vi "ATE_spoldrx_cal_at_IF.vi"() -> ()   [LabVIEW 2012]
doc: "Use this template to build a producer/consumer design pattern with events to produce queue items. Use this design pattern instead of the User Interface Event Handler pattern for user interfaces when you want to execute code asynchronously in response to an event without slowing the user interface responsiveness."
uses:
  Rvp8PowerData.ctl
  <vilib>/Analysis/NI_AALPro.lvlib
panel:
  in  "ABORT":bool
  in  "READY":bool
  out "Instructions":string="rvp8 calibration vi\n\n1 - Disable or turn off transmitter\n2 - Stow Antenna (point vertically)\n3 - Start the labview program by clicking the Run arrow\n     (left most button under  drop down menues)\n     start cycle time about 35 seconds\n3 - Wait for the red 'BUSY' light to change to green 'READY'\n     The 'active' controls on the control tab are the 'TsPring/TsGrabber'\n     and the 'Start dBm', 'Step Size' and 'Steps' controls \n4 - Calibrate with the red  'Calibrate' button\n      calibration cycle time is about 5 minutes\n5 - Calibration cycle can be aborted with the 'Abort Cal' button which\n     is visable only during the cal cycle\n6 - exit the program with the red 'EXIT' button\n      exit cycle time about 20 seconds\n\nHints:\nWait for the green 'READY' light before clicking buttons"
  out "70dB\nAttenuators":bool[](array[boolean])
  out "70 Verfied":bool
  out "121dB\nAttenuators":bool[](array[boolean])
  out "121 Verified":bool
  in  "Configuration 1":bool
  out "Cal Output File":path
  out "Cal differences":cluster{dbl[], dbl[]}[](graph)
  out "drx calibration":cluster{dbl[], dbl[]}[](graph)
  out "Cal file name":string
  in  "Cal data directory":string="/home/spol/projDir/data/cal/ate/drx_cal"
  in  "Set SigGen":bool
  in  "Initialize":bool
  in  "70 dB":bool
  in  "121 dB":bool
  in  "Switches":bool
  in  "Calibrate":bool
  in  "Stop":bool
  in  "ATE TABS":enum32{"Status", "Controls"}(tab)=enum."Controls"
  out "ATE Switch Status":T1
  out "drx Power":T2 {"time" format="%<%H:%M:%S\n%Y/%m/%d>T"}
  out "Signal Generator Status":T3={"Frequency (GHz)"=0.0, "RF Power (dBm)"=0.0, "RF Power"=TRUE} {"RF Power (dBm)" format="%.2g"}
  in  "Start dBm":dbl=-14.0 min=-100.0 max=14.0 step=1.0
  in  "Steps":i32=64
  in  "Steps Size":dbl=2.0 min=0.1 max=10.0 step=0.1 format="%.1g"
  in  "121 dB Atten":i32=121 min=0 max=121 step=1
  in  "70 dB Attn":i32=70 min=0 max=70 step=10
  in  "ATE Switches":T4={"Reversing Switch"=enum."Normal Function", "IO Switch #1 Input"=enum."NONE", "IO Switch #1 Output"=enum."NONE", "IO Switch #2 Input"=enum."NONE", "IO Switch #2 Output"=enum."NONE", "Signal Out Input"=enum."NONE", "Signal Out Output"=enum."NONE", "Signal Source Input"=enum."NONE", "Signal Source Output"=enum."NONE", "Power Meter Switch Input"=enum."NONE", "Pouer Meter Switch Output"=enum."NONE", "Amplifier Switch"=enum."Include Amp"}
  out "P-State":string
  out "C-State":string
  in  "BUSY":bool
  # "ATE drx cal Program"
  # "10 dB"
  # "20 dB"
  # "40 dB"
  # "1 dB"
  # "2 dB"
  # "4 dB"
  # "4 dB"
  # "10 dB"
  # "20 dB"
  # "40 dB"
  # "40 dB"
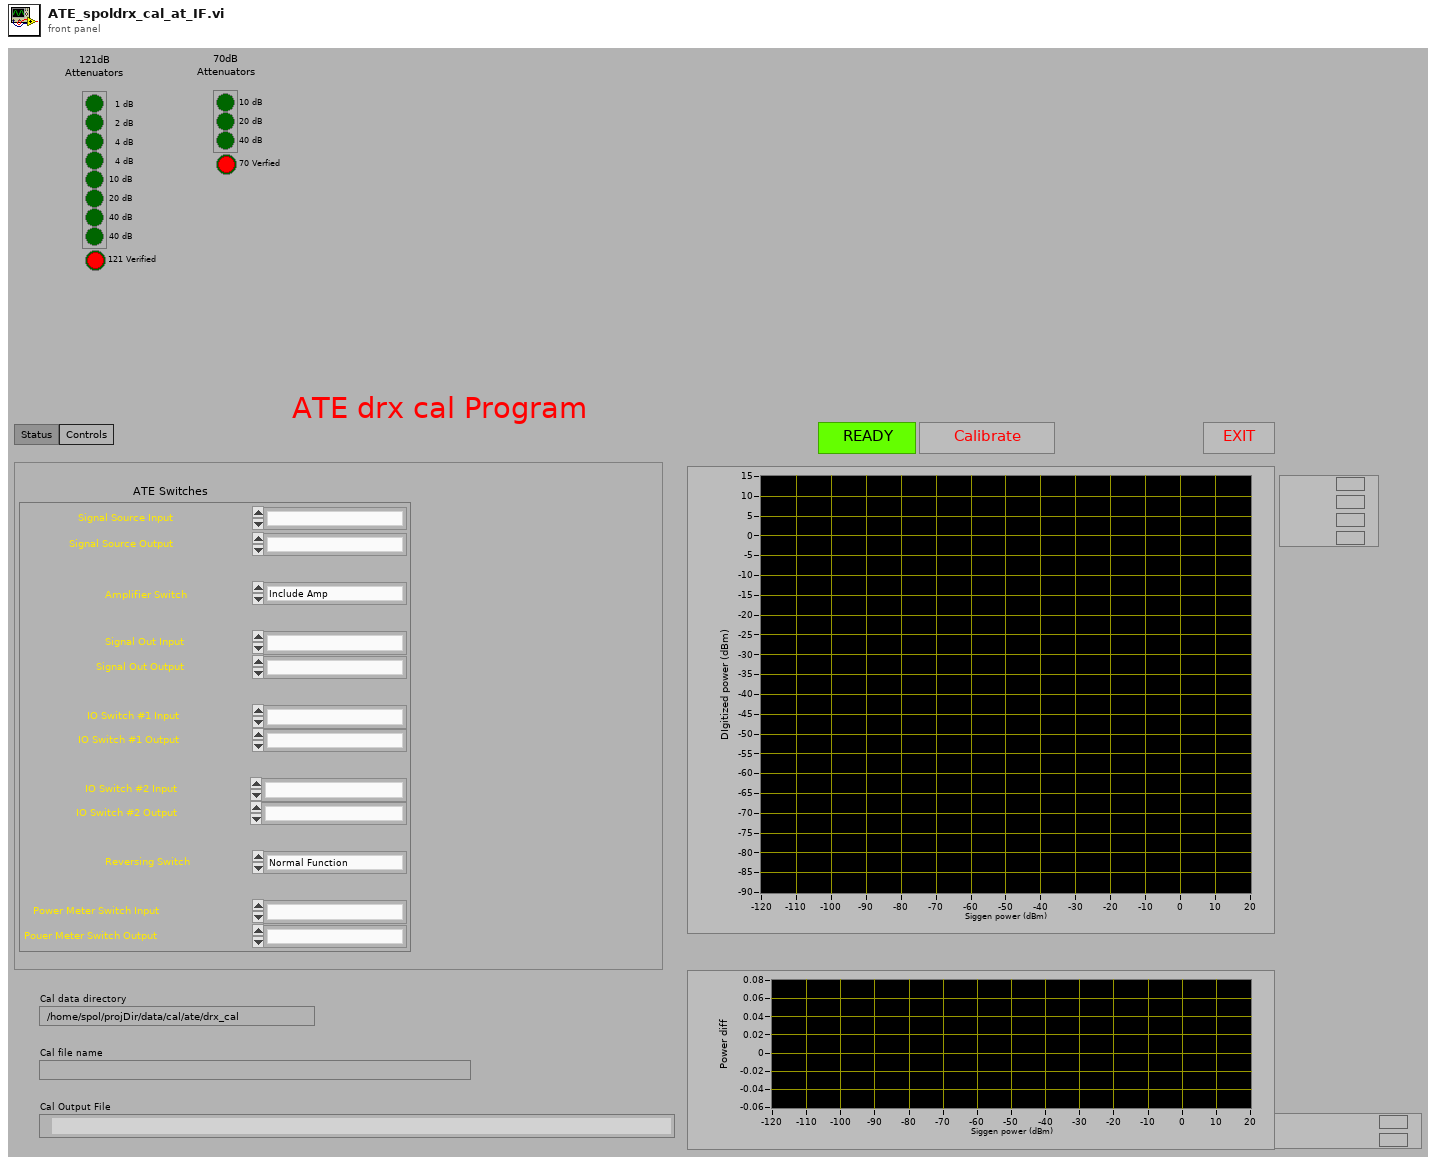
[diagram p1: front panel]
types:
  T1 = cluster{"Reversing Switch ":bool, "IO Switch #1":bool, "IO Switch #2":bool, "Signal Out":bool, "Signal Source":bool, "Power Meter":bool, "Amp By Pass":bool}
  T2 = typedef "Rvp8PowerData.ctl" = cluster{"success":bool, "time":dbl, "el":dbl, "az":dbl, "dbm0":dbl, "dbm1":dbl, "dbmHc":dbl, "dbmHx":dbl, "dbmVc":dbl, "dbmVx":dbl}
  T3 = cluster{"Frequency (GHz)":dbl, "RF Power (dBm)":dbl, "RF Power":bool}
  T4 = cluster{"Reversing Switch":enum16{"Normal Function", "Reversing Function"}, "IO Switch #1 Input":enum16{"NONE", "AHR (J2)", "Splitter", "Signal Out Switch (S3)", "Reversing Switch"}, "IO Switch #1 Output":enum16{"NONE", "AHR (J2)", "Delay Device (S4)", "Power Meter Switch (S5)", "Reversing Switch"}, "IO Switch #2 Input":enum16{"NONE", "AVR (J3)", "Splitter", "Signal Out Switch (S3)", " 2W Term (TM1)", "Reversing Switch"}, "IO Switch #2 Output":enum16{"NONE", "AVR (J3)", "Signal Out Switch (S3)", "Power Meter Switch (S5)", "Reversing Switch", "2W Term (TM1)"}, "Signal Out Input":enum16{"NONE", "Amp Bypass Switch (S6)", "IO Switch #1 (S1)", "IO Switch #2 (S2)", "2W Term (TM3)"}, "Signal Out Output":enum16{"NONE", "2 Watt Term (TM3)", "Splitter", "Power Meter Switch (S5)"}, "Signal Source Input":enum16{"NONE", "Delay Device", "Signal Generator (J7)", "Inside Noise Box NF (J5)", "2W Term (TM3)"}, "Signal Source Output":enum16{"NONE", "Amp Bypass Switch", "Test Pulse Generator", "Power Meter Switch (S5)"}, "Power Meter Switch Input":enum16{"NONE", "IO Switch #1 (S1)", "Signal Source Switch (S4)", "Signal Out Switch (S3)", "IO Switch #2 (S2)", "TXH-TXV Switch (J8)"}, "Pouer Meter Switch Output":enum16{"NONE", "Power Meter (J6)"}, "Amplifier Switch":enum16{"Bypass Amp", "Include Amp"}}
  T5 = cluster{"Frequency (GHz)":dbl, "RF Power (dBm)":dbl, "RF ON/OFF":bool}
  T6 = enum16{"open", "replace", "create", "open or create", "replace or create", "replace or create with confirmation"}
  T7 = typedef "drxPowerData.ctl" = cluster{"success":bool, "time":dbl, "el":dbl, "az":dbl, "dbm0":dbl, "dbm1":dbl, "dbmHc":dbl, "dbmHx":dbl, "dbmVc":dbl, "dbmVx":dbl}
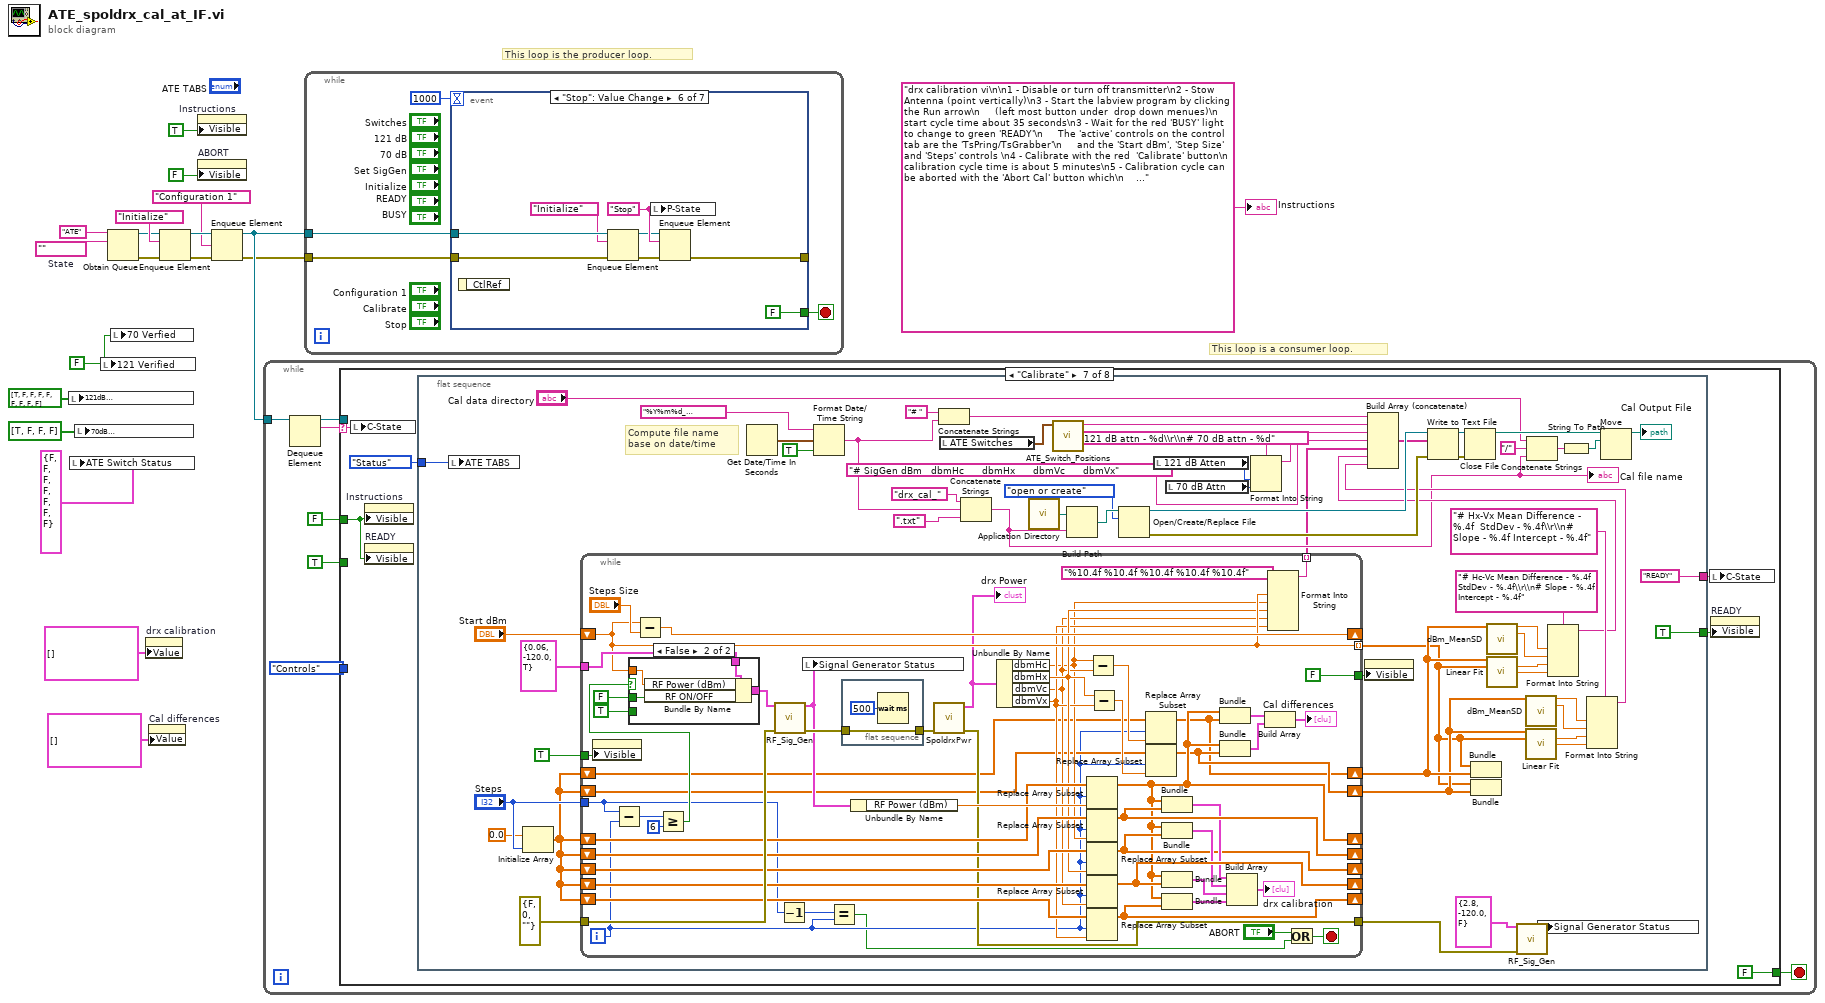
[diagram p0: block diagram]
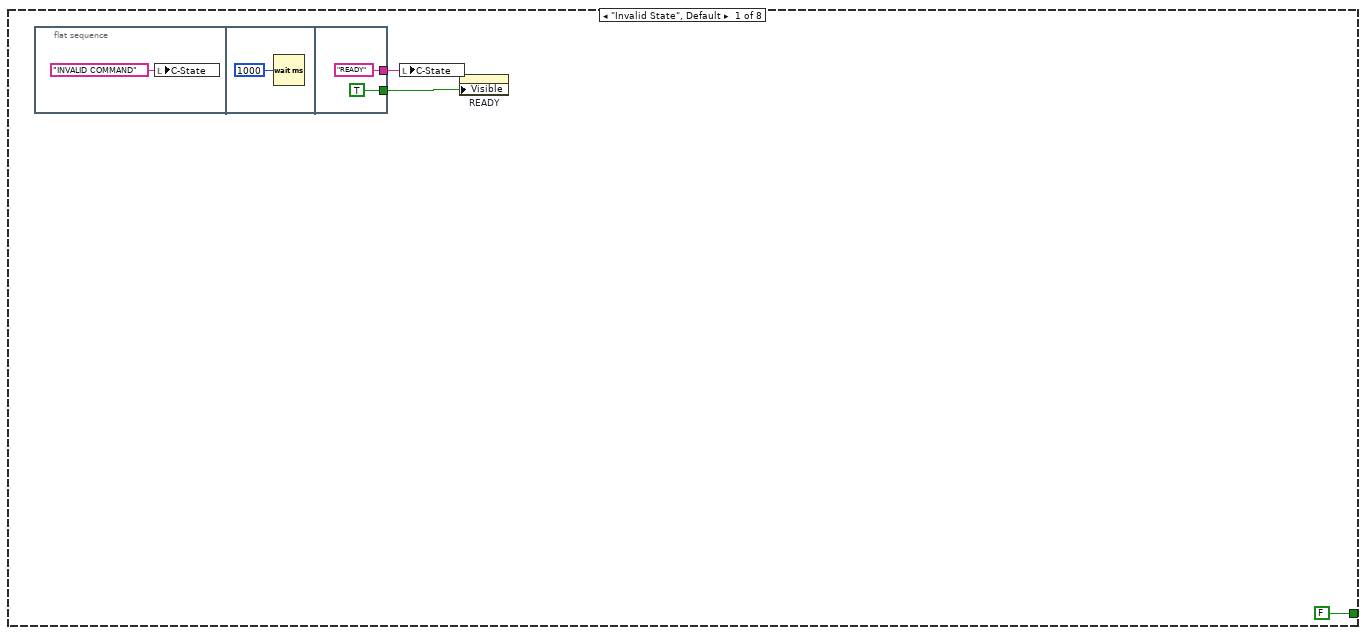
[diagram p2: hidden frame]
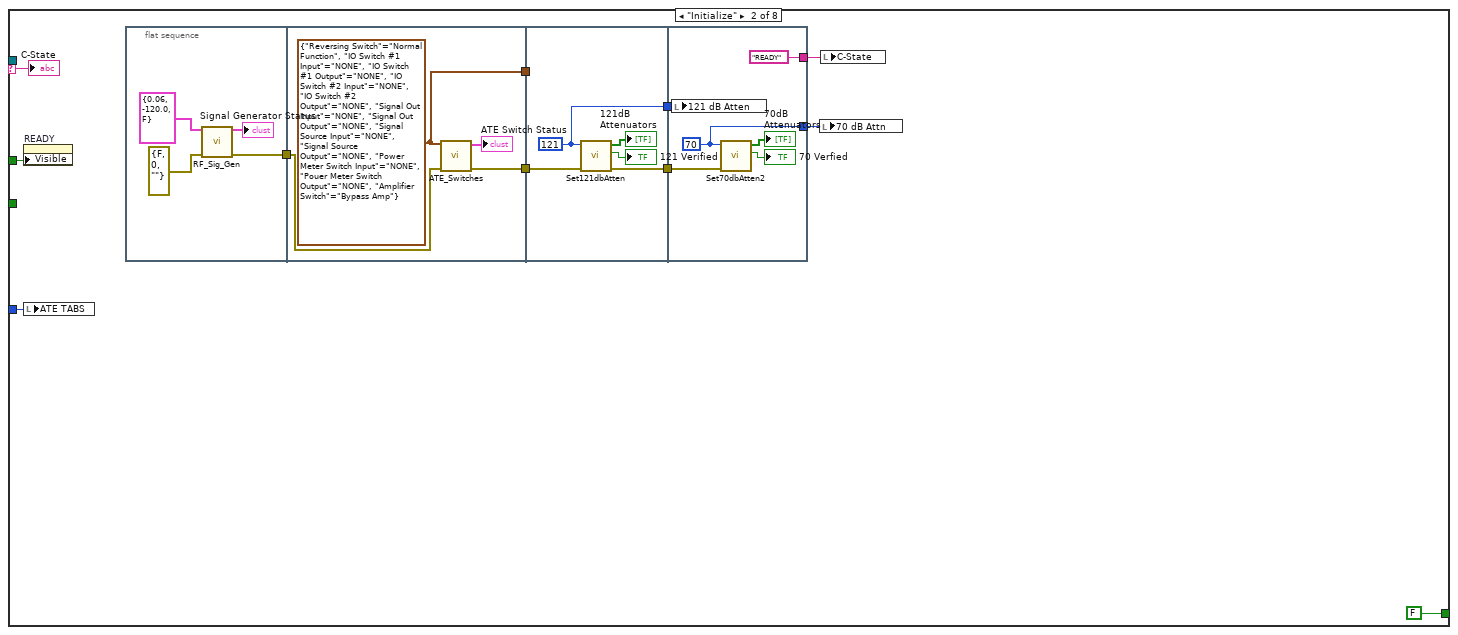
[diagram p3: hidden frame]
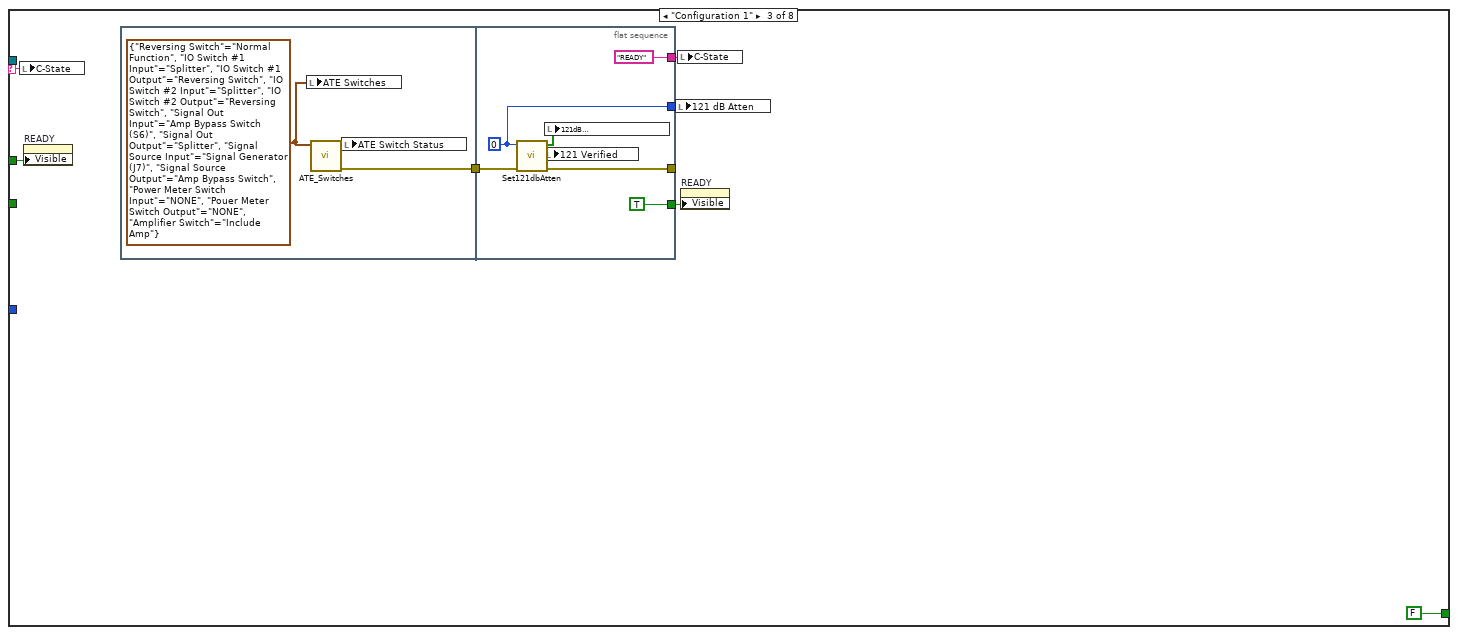
[diagram p4: hidden frame]
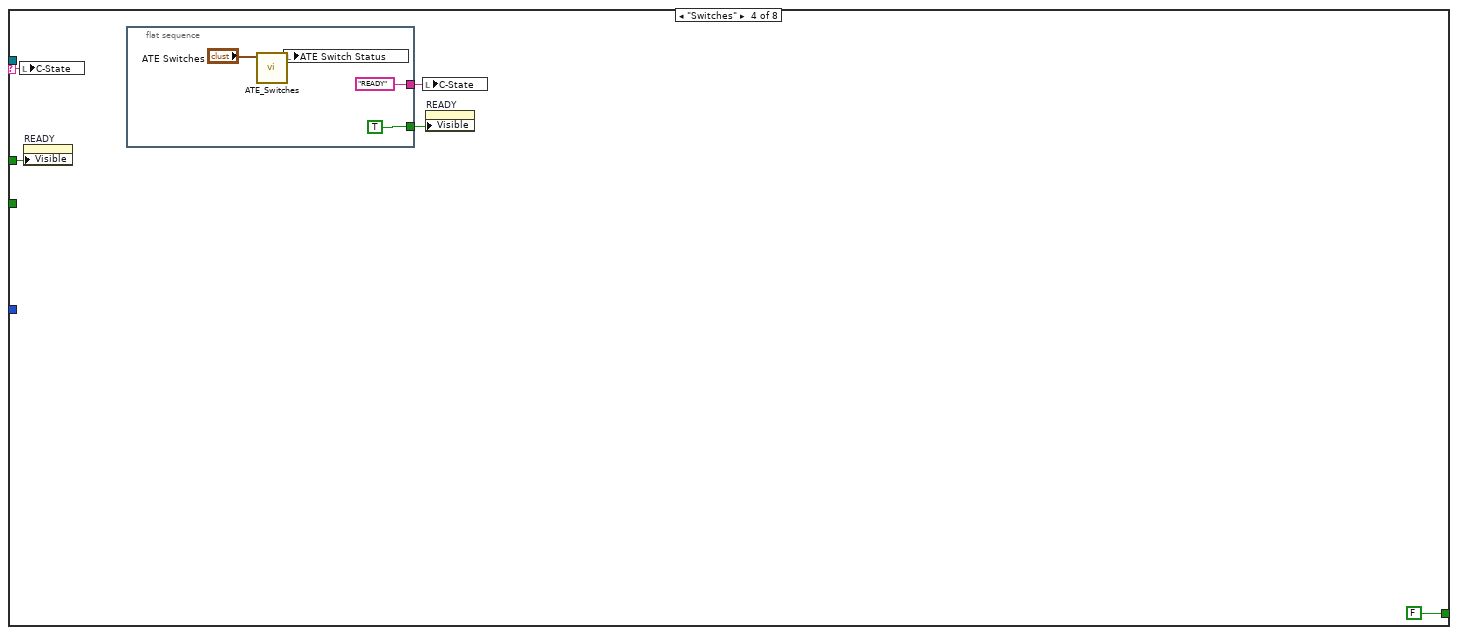
[diagram p5: hidden frame]
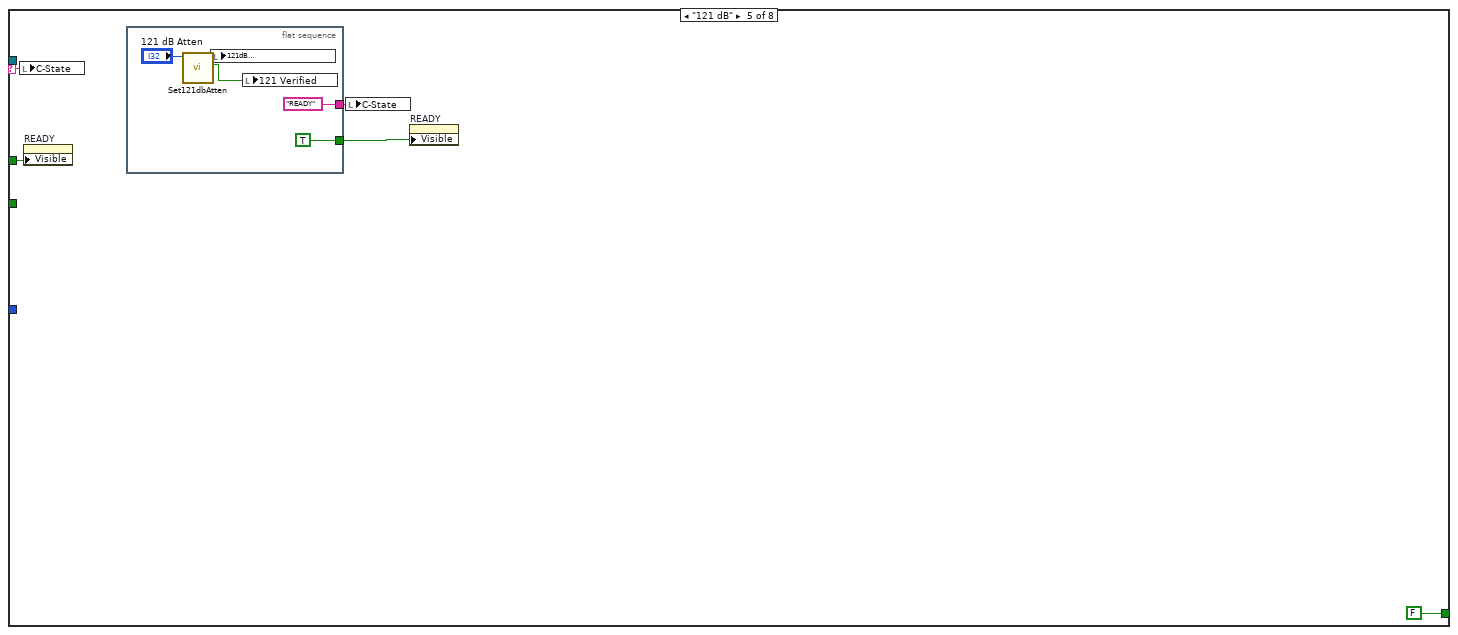
[diagram p6: hidden frame]
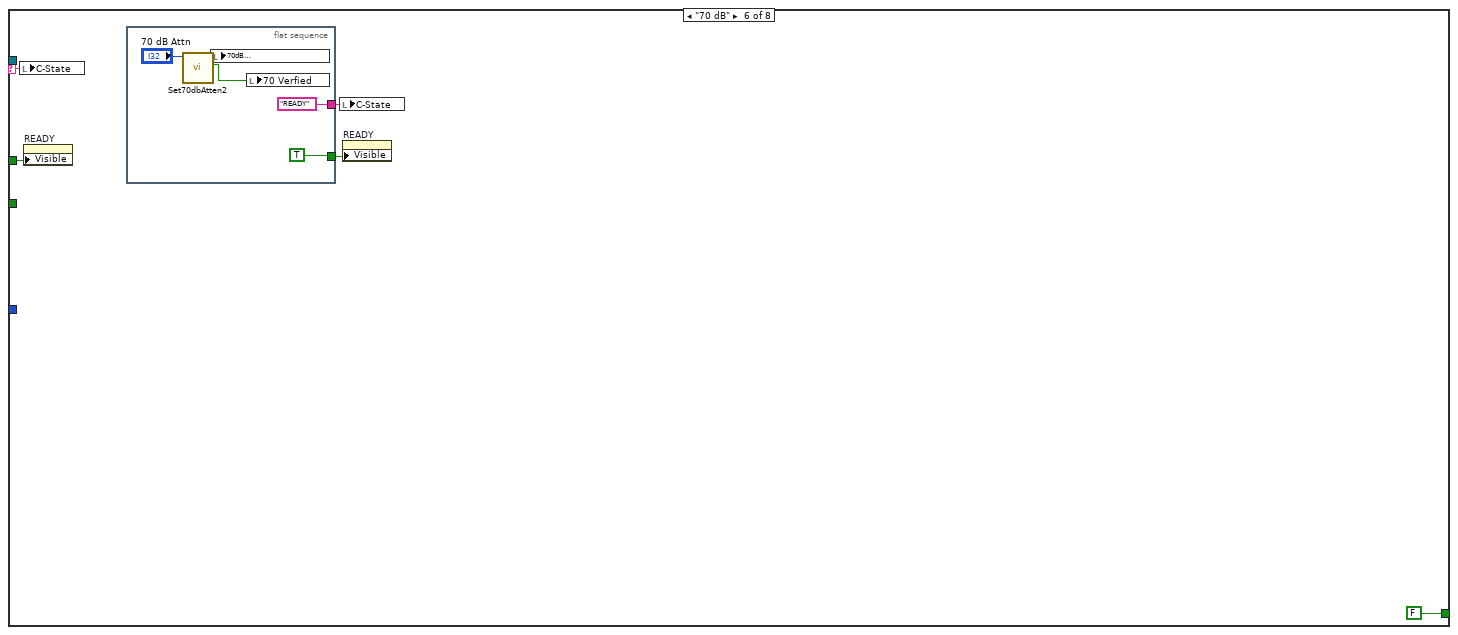
[diagram p7: hidden frame]
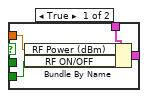
[diagram p8: hidden frame]
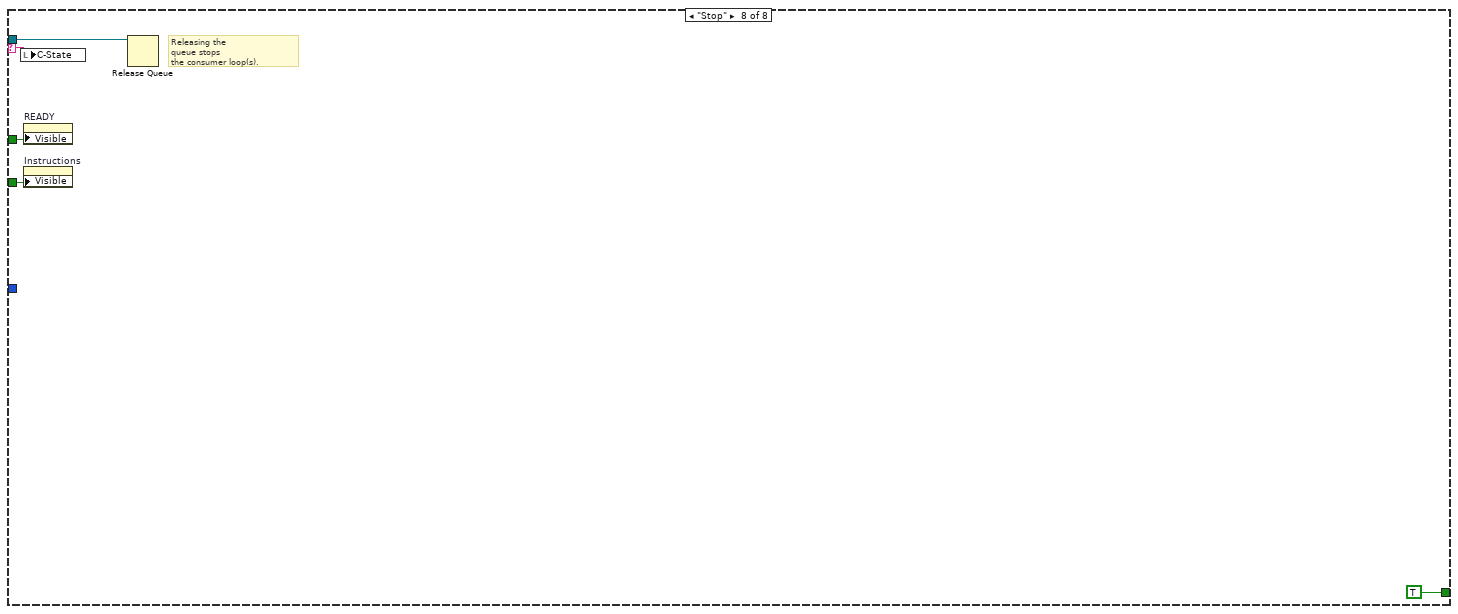
[diagram p9: hidden frame]
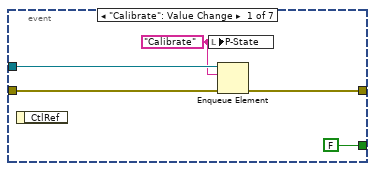
[diagram p10: hidden frame]
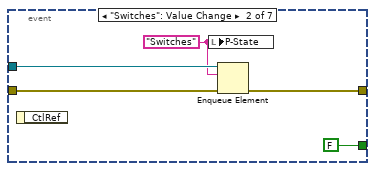
[diagram p11: hidden frame]
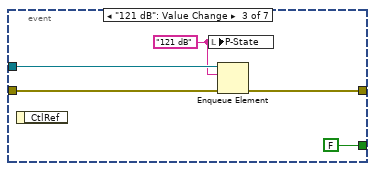
[diagram p12: hidden frame]
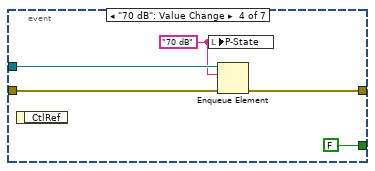
[diagram p13: hidden frame]
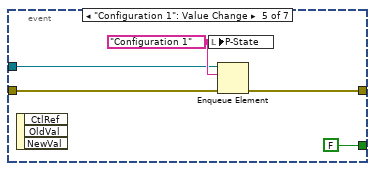
[diagram p14: hidden frame]
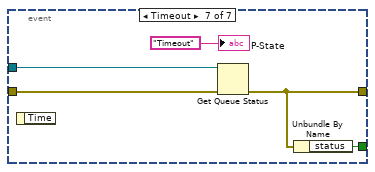
[diagram p15: hidden frame]
diagram:
  w4 = FALSE ("70 Verfied")
  w19 = ""  # State
  # "This loop is the producer loop."
  # "This loop is a consumer loop."
  n1 = local write "121dB\nAttenuators"(bool[] [TRUE, FALSE, FALSE, FALSE, FALSE, FALSE, FALSE, FALSE, FALSE] ("121dB\nAttenuators")) -> ()
  n2 = local write "ATE Switch Status"(T1 {"Reversing Switch "=FALSE, "IO Switch #1"=FALSE, "IO Switch #2"=FALSE, "Signal Out"=FALSE, "Signal Source"=FALSE, "Power Meter"=FALSE, "Amp By Pass"=FALSE} ("ATE Switch Status")) -> ()
  n3 = local write "70dB\nAttenuators"(bool[] [TRUE, FALSE, FALSE, FALSE] ("70dB\nAttenuators")) -> ()
  n4 = local write "121 Verified"(w4) -> ()
  n5 = Obtain Queue(name (unnamed)="ATE", element data type=w19) -> (queue out=w16:refnum<queue>, error out=w14:errorcluster)  [unwired: 3 in, 1 out]
  n6 = local write "70 Verfied"(w4) -> ()
  n7 = property on="drx calibration" class="XYGraph (strict)"("Value"=cluster{dbl[], dbl[]}[] [] ("drx calibration")) -> ()  [unwired: 2 in, 2 out]
  n8 = property on="Cal differences" class="XYGraph (strict)"("Value"=cluster{dbl[], dbl[]}[] [] ("Cal differences")) -> ()  [unwired: 2 in, 2 out]
  n9 = Enqueue Element(queue=w16, element="Initialize", error in (no error)=w14) -> (queue out=w15:refnum<queue>, error out=w9:errorcluster)  [unwired: 1 in, 1 out]
  n10 = property on="Instructions" class="Str"("Visible"=TRUE) -> ()  [unwired: 2 in, 2 out]
  n11 = property on="ABORT" class="Bool"("Visible"=FALSE) -> ()  [unwired: 2 in, 2 out]
  n12 = Enqueue Element(queue=w15, element="Configuration 1", error in (no error)=w9) -> (queue out=w10:refnum<queue>, error out=w8:errorcluster)  [unwired: 1 in, 1 out]
  n13 = while {
    tunnel: w10 -> [w26]
    stop <- w23 stop-if-true
    n14 = Dequeue Element(queue=w26) -> (queue out=w24:refnum<queue>, element=w25:string)  [unwired: 2 in, 2 out]
    n15 = case shown="\"Calibrate\"" w25 {
      selector: w25 -> [_ w43 w66 w85 w93 w103 w114 w244]
      tunnel: w24 -> [_ _ _ _ _ _ _ w243]
      tunnel: [FALSE FALSE FALSE FALSE FALSE FALSE FALSE TRUE] -> w23
      tunnel: FALSE ("Visible") -> [_ w35 w65 w82 w91 w101 w112 w242]
      tunnel: TRUE ("Visible") -> [_ _ _ _ _ _ _ w241]
      tunnel: enum32{"Status", "Controls"}."Controls" ("ATE TABS") -> [_ w34 _ _ _ _ _ _]
      frame "Invalid State", Default {
        n16 = flat-sequence {
          tunnel: ["READY" ("element")] -> w28
          tunnel: [TRUE ("Visible")] -> w27
          frame #0 {
            n17 = local write "C-State"("INVALID COMMAND" ("C-State")) -> ()
          }
          frame #1 {
            n18 = Wait (ms)(milliseconds to wait=u32 1000) -> ()  [unwired: 1 out]
          }
          frame #2 {
          }
        }
        n19 = local write "C-State"(w28) -> ()
        n20 = property on="READY" class="Bool"("Visible"=w27) -> ()  [unwired: 2 in, 2 out]
      }
      frame "Initialize" {
        n21 = property on="READY" class="Bool"("Visible"=w35) -> ()  [unwired: 2 in, 2 out]
        n22 = local write "ATE TABS"(w34) -> ()
        n23 = flat-sequence {
          tunnel: [w45] -> w37
          tunnel: [w50] -> w40
          tunnel: w37 -> [w51]
          tunnel: [w49] -> w36
          tunnel: w40 -> [w56]
          tunnel: [w55] -> w41
          tunnel: [w54] -> w39
          tunnel: w36 -> [_]
          tunnel: ["READY" ("element")] -> w42
          tunnel: w41 -> [w62]
          tunnel: w39 -> [w60]
          tunnel: [w59] -> w38
          frame #0 {
            n24 = call "RF_Sig_Gen.vi"("Signal Generator Control"=T5 {"Frequency (GHz)"=0.06, "RF Power (dBm)"=-120.0, "RF ON/OFF"=FALSE}, "error in"=errorcluster {"status"=FALSE, "code"=0, "source"=""}) -> ("Signal Generator Status"=→"Signal Generator Status":T3, "Sig Gen Errors"=w45:errorcluster)  [unwired: 12 in]
          }
          frame #1 {
            w49 = T4 {"Reversing Switch"=enum."Normal Function", "IO Switch #1 Input"=enum."NONE", "IO Switch #1 Output"=enum."NONE", "IO Switch #2 Input"=enum."NONE", "IO Switch #2 Output"=enum."NONE", "Signal Out Input"=enum."NONE", "Signal Out Output"=enum."NONE", "Signal Source Input"=enum."NONE", "Signal Source Output"=enum."NONE", "Power Meter Switch Input"=enum."NONE", "Pouer Meter Switch Output"=enum."NONE", "Amplifier Switch"=enum."Bypass Amp"} ("ATE Switches")
            n25 = call "ATE_Switches.vi"("error in"=w51, "ATE Switches"=w49) -> ("Switch Errors"=w50:errorcluster, "ATE Switch Status"=→"ATE Switch Status":T1)  [unwired: 8 in]
          }
          frame #2 {
            w54 = 121 ("Attenuation (dB)")
            n26 = call "Set121dbAtten.vi"("error in (no error)"=w56, "Attenuation (dB)"=w54) -> ("error out"=w55:errorcluster, "Verfied"=→"121 Verified":bool, "Active Attenuators"=→"121dB\nAttenuators":bool[])  [unwired: 7 in]
          }
          frame #3 {
            w59 = 70 ("Attenuation (dB)")
            n27 = local write "121 dB Atten"(w60) -> ()
            n28 = call "Set70dbAtten2.vi"("error in (no error)"=w62, "Attenuation (dB)"=w59) -> ("Verfied"=→"70 Verfied":bool, "Active Attenuators"=→"70dB\nAttenuators":bool[])  [unwired: 7 in, 1 out]
          }
        }
        n29 = local write "70 dB Attn"(w38) -> ()
        n30 = local write "C-State"(w42) -> ()
        "C-State" <- w43
      }
      frame "Configuration 1" {
        n31 = local write "C-State"(w66) -> ()
        n32 = property on="READY" class="Bool"("Visible"=w65) -> ()  [unwired: 2 in, 2 out]
        n33 = flat-sequence {
          tunnel: [w73] -> w69
          tunnel: w69 -> [w80]
          tunnel: [w75] -> w68
          tunnel: ["READY" ("element")] -> w67
          tunnel: [w78] -> _
          tunnel: [TRUE ("Visible")] -> w64
          frame #0 {
            w71 = T4 {"Reversing Switch"=enum."Normal Function", "IO Switch #1 Input"=enum."Splitter", "IO Switch #1 Output"=enum."Reversing Switch", "IO Switch #2 Input"=enum."Splitter", "IO Switch #2 Output"=enum."Reversing Switch", "Signal Out Input"=enum."Amp Bypass Switch (S6)", "Signal Out Output"=enum."Splitter", "Signal Source Input"=enum."Signal Generator (J7)", "Signal Source Output"=enum."Amp Bypass Switch", "Power Meter Switch Input"=enum."NONE", "Pouer Meter Switch Output"=enum."NONE", "Amplifier Switch"=enum."Include Amp"} ("ATE Switches")
            n34 = local write "ATE Switches"(w71) -> ()
            n35 = call "ATE_Switches.vi"("ATE Switches"=w71) -> ("Switch Errors"=w73:errorcluster, "ATE Switch Status"=w72:T1)  [unwired: 9 in]
            n36 = local write "ATE Switch Status"(w72) -> ()
          }
          frame #1 {
            w75 = 0 ("Attenuation (dB)")
            n37 = call "Set121dbAtten.vi"("error in (no error)"=w80, "Attenuation (dB)"=w75) -> ("error out"=w78:errorcluster, "Verfied"=w76:bool, "Active Attenuators"=w77:bool[])  [unwired: 7 in]
            n38 = local write "121 Verified"(w76) -> ()
            n39 = local write "121dB\nAttenuators"(w77) -> ()
          }
        }
        n40 = local write "121 dB Atten"(w68) -> ()
        n41 = local write "C-State"(w67) -> ()
        n42 = property on="READY" class="Bool"("Visible"=w64) -> ()  [unwired: 2 in, 2 out]
      }
      frame "Switches" {
        n43 = local write "C-State"(w85) -> ()
        n44 = property on="READY" class="Bool"("Visible"=w82) -> ()  [unwired: 2 in, 2 out]
        n45 = flat-sequence {
          tunnel: ["READY" ("element")] -> w83
          tunnel: [TRUE ("Visible")] -> w81
          frame #0 {
            n46 = call "ATE_Switches.vi"("ATE Switches"="ATE Switches") -> ("ATE Switch Status"=w88:T1)  [unwired: 9 in, 1 out]
            n47 = local write "ATE Switch Status"(w88) -> ()
          }
        }
        n48 = local write "C-State"(w83) -> ()
        n49 = property on="READY" class="Bool"("Visible"=w81) -> ()  [unwired: 2 in, 2 out]
      }
      frame "121 dB" {
        n50 = local write "C-State"(w93) -> ()
        n51 = property on="READY" class="Bool"("Visible"=w91) -> ()  [unwired: 2 in, 2 out]
        n52 = flat-sequence {
          tunnel: ["READY" ("element")] -> w92
          tunnel: [TRUE ("Visible")] -> w90
          frame #0 {
            n53 = call "Set121dbAtten.vi"("Attenuation (dB)"="121 dB Atten") -> ("Verfied"=w96:bool, "Active Attenuators"=w98:bool[])  [unwired: 8 in, 1 out]
            n54 = local write "121dB\nAttenuators"(w98) -> ()
            n55 = local write "121 Verified"(w96) -> ()
          }
        }
        n56 = local write "C-State"(w92) -> ()
        n57 = property on="READY" class="Bool"("Visible"=w90) -> ()  [unwired: 2 in, 2 out]
      }
      frame "70 dB" {
        n58 = local write "C-State"(w103) -> ()
        n59 = property on="READY" class="Bool"("Visible"=w101) -> ()  [unwired: 2 in, 2 out]
        n60 = flat-sequence {
          tunnel: ["READY" ("element")] -> w102
          tunnel: [TRUE ("Visible")] -> w100
          frame #0 {
            n61 = call "Set70dbAtten2.vi"("Attenuation (dB)"="70 dB Attn") -> ("Verfied"=w106:bool, "Active Attenuators"=w108:bool[])  [unwired: 8 in, 1 out]
            n62 = local write "70dB\nAttenuators"(w108) -> ()
            n63 = local write "70 Verfied"(w106) -> ()
          }
        }
        n64 = local write "C-State"(w102) -> ()
        n65 = property on="READY" class="Bool"("Visible"=w100) -> ()  [unwired: 2 in, 2 out]
      }
      frame "Calibrate" {
        n66 = local write "C-State"(w114) -> ()
        n67 = property on="Instructions" class="Str"("Visible"=w112) -> ()  [unwired: 2 in, 2 out]
        n68 = property on="READY" class="Bool"("Visible"=w112) -> ()  [unwired: 2 in, 2 out]
        n69 = flat-sequence {
          tunnel: ["READY" ("element")] -> w113
          tunnel: [TRUE ("Visible")] -> w111
          tunnel: enum32{"Status", "Controls"}."Status" ("ATE TABS") -> [w121]
          frame #0 {
            # "Compute file name base on date/time"
            n70 = local write "ATE TABS"(w121) -> ()
            n71 = Initialize Array(0.0 ("element"), "Steps") -> (w120:dbl[])
            n72 = while {
              shift-right: [w224] -> _
              shift-left: "Start dBm" -> [w222]
              tunnel: errorcluster {"status"=FALSE, "code"=0, "source"=""} ("error out") -> [w216]
              tunnel: [w222] -> w123 mode=indexing
              tunnel: [w230] -> w126 mode=indexing
              tunnel: T5 {"Frequency (GHz)"=0.06, "RF Power (dBm)"=-120.0, "RF ON/OFF"=TRUE} ("Signal Generator Control") -> [w229]
              tunnel: [w194] -> w156
              tunnel: "Steps" -> [w179]
              shift-right: [w193] -> _
              shift-left: w120 -> [w208]
              shift-right: [w205] -> _
              shift-left: w120 -> [w212]
              shift-right: [w195] -> _
              shift-left: w120 -> [w213]
              shift-right: [w207] -> _
              shift-left: w120 -> [w214]
              shift-right: [w206] -> _
              shift-left: w120 -> [w215]
              shift-right: [w189] -> w148
              shift-left: w120 -> [w187]
              shift-right: [w190] -> w147
              shift-left: w120 -> [w188]
              tunnel: [FALSE ("Visible")] -> w119
              tunnel: TRUE ("Visible") -> [w176]
              i -> [w181]
              stop <- w183 stop-if-true
              n73 = property on="ABORT" class="Bool"("Visible"=w176) -> ()  [unwired: 2 in, 2 out]
              n74 = Subtract(x=w179, y=w181) -> (x-y=w217:i32)
              n75 = Subtract(x=w222, y="Steps Size") -> (x-y=w224:dbl)
              n76 = Greater Or Equal?(x=w217, y=6) -> (x >= y?=w219:bool)
              n77 = case shown="False" w219 {
                tunnel: w229 -> [w234 w238]
                tunnel: [w233 w237] -> w225
                tunnel: w222 -> [w232 w236]
                tunnel: FALSE ("70 Verfied") -> [_ w235]
                tunnel: TRUE ("70 Verfied") -> [w231 _]
                frame True {
                  n78 = Bundle By Name(cluster=w234, "RF Power (dBm)"=w232, "RF ON/OFF"=w231) -> (w233:T5)
                }
                frame False {
                  n79 = Bundle By Name(cluster=w238, "RF Power (dBm)"=w236, "RF ON/OFF"=w235) -> (w237:T5)
                }
              }
              n80 = call "RF_Sig_Gen.vi"("Signal Generator Control"=w225, "error in"=w216) -> ("Signal Generator Status"=w210:T3, "Sig Gen Errors"=w228:errorcluster)  [unwired: 12 in]
              n81 = Decrement(x=w179) -> (x-1=w180:i32)
              n82 = local write "Signal Generator Status"(w210) -> ()
              n83 = Equal?(x=w180, y=w181) -> (x = y?=w178:bool)
              n84 = flat-sequence {
                tunnel: w228 -> [w240]
                tunnel: [w240] -> w227
                frame #0 {
                  n85 = Wait (ms)(milliseconds to wait=u32 500) -> ()  [unwired: 1 out]
                }
              }
              n86 = Unbundle By Name(w210) -> ("RF Power (dBm)"=w209:dbl)
              n87 = call "SpoldrxPwr.vi"("error in (no error)"=w227) -> ("Comm error"=w194:errorcluster, "drx_power"=w211:T7)  [unwired: 7 in, 2 out]
              "drx Power" <- w211
              n88 = Unbundle By Name(w211) -> ("dbmHc"=w196:dbl, "dbmHx"=w199:dbl, "dbmVc"=w197:dbl, "dbmVx"=w198:dbl)
              n89 = Replace Array Subset(array=w208, new element=w209, index=w181) -> (w193:dbl[])
              n90 = Replace Array Subset(array=w212, new element=w196, index=w181) -> (w205:dbl[])
              n91 = Replace Array Subset(array=w213, new element=w199, index=w181) -> (w195:dbl[])
              n92 = Replace Array Subset(array=w214, new element=w197, index=w181) -> (w207:dbl[])
              n93 = Replace Array Subset(array=w215, new element=w198, index=w181) -> (w206:dbl[])
              n94 = Subtract(x=w196, y=w197) -> (x-y=w192:dbl)
              n95 = Subtract(x=w199, y=w198) -> (x-y=w191:dbl)
              n96 = Replace Array Subset(array=w187, new element=w192, index=w181) -> (w189:dbl[])
              n97 = Replace Array Subset(array=w188, new element=w191, index=w181) -> (w190:dbl[])
              n98 = Bundle(w193, w205) -> (w201:cluster{dbl[], dbl[]})  [unwired: 1 in]
              n99 = Bundle(w193, w195) -> (w202:cluster{dbl[], dbl[]})  [unwired: 1 in]
              n100 = Bundle(w193, w207) -> (w203:cluster{dbl[], dbl[]})  [unwired: 1 in]
              n101 = Bundle(w193, w206) -> (w204:cluster{dbl[], dbl[]})  [unwired: 1 in]
              n102 = Bundle(w193, w189) -> (w185:cluster{dbl[], dbl[]})  [unwired: 1 in]
              n103 = Bundle(w193, w190) -> (w186:cluster{dbl[], dbl[]})  [unwired: 1 in]
              n104 = Build Array(w201, w202, w203, w204) -> (→"drx calibration":cluster{dbl[], dbl[]}[])
              n105 = Build Array(w185, w186) -> (→"Cal differences":cluster{dbl[], dbl[]}[])
              n106 = Format Into String(format string="%10.4f %10.4f %10.4f %10.4f %10.4f", w222, w196, w199, w197, w198) -> (resulting string=w230:string)  [unwired: 2 in, 1 out]
              n107 = Or(x="ABORT", y=w178) -> (x .or. y?=w183:bool)
            }
            n108 = Get Date/Time In Seconds() -> (seconds since 1Jan1904=w170:timestamp)
            n109 = Format Date/Time String(time format string (%c)="%Y%m%d_%H%M%S", seconds (now)=w170, UTC format=TRUE) -> (date/time string=w128:string)
            n110 = Concatenate Strings("# " ("string"), w128) -> (w141:string)
            n111 = local read "ATE Switches"() -> (w134:T4)
            n112 = Concatenate Strings("drx_cal_", w128, ".txt") -> (w127:string)
            "Cal file name" <- w127
            n113 = call <vilib>:"Application Directory.vi"() -> ("Application Directory"=w132:path)
            n114 = call "ATE_Switch_Positions.vi"("ATE Switches"=w134) -> ("ATE Switch/Position"=w140:string)  [unwired: 10 in]
            n115 = Build Path(base path=w132, name or relative path=w127) -> (appended path=w167:path)
            n116 = Open/Create/Replace File(file path (use dialog)=w167, operation (0:open)=T6."open or create") -> (refnum out=w166:refnum<file>, error out=w165:errorcluster)  [unwired: 4 in, 1 out]
            n117 = local read "121 dB Atten"() -> (w153:i32)
            n118 = local read "70 dB Attn"() -> (w152:i32)
            n119 = Format Into String(format string="# 121 dB attn - %d\\r\\n# 70 dB attn - %d", w153, w152) -> (resulting string=w139:string)  [unwired: 2 in, 1 out]
            n120 = property on="ABORT" class="Bool"("Visible"=w119) -> ()  [unwired: 2 in, 2 out]
            n121 = Bundle(w123, w148) -> ()  [unwired: 1 in, 1 out]
            n122 = Bundle(w123, w147) -> ()  [unwired: 1 in, 1 out]
            n123 = call "dBm_MeanSD.vi"("dBm array"=w148) -> ("dBm mean"=w151:dbl, "Std Dev"=w116:dbl)  [unwired: 13 in]
            n124 = call <vilib>:"Linear Fit.vi"("Y"=w148, "X"=w123) -> ("slope"=w150:dbl, "intercept"=w149:dbl)  [unwired: 9 in, 3 out]
            n125 = call "RF_Sig_Gen.vi"("Signal Generator Control"=T5 {"Frequency (GHz)"=2.8, "RF Power (dBm)"=-120.0, "RF ON/OFF"=FALSE}, "error in"=w156) -> ("Signal Generator Status"=w157:T3)  [unwired: 12 in, 1 out]
            n126 = call "dBm_MeanSD.vi"("dBm array"=w147) -> ("dBm mean"=w146:dbl, "Std Dev"=w117:dbl)  [unwired: 13 in]
            n127 = call <vilib>:"Linear Fit.vi"("Y"=w147, "X"=w123) -> ("slope"=w145:dbl, "intercept"=w144:dbl)  [unwired: 9 in, 3 out]
            n128 = Concatenate Strings("Cal data directory", "/" ("string"), w127) -> (w161:string)
            n129 = local write "Signal Generator Status"(w157) -> ()
            n130 = Format Into String(format string="# Hc-Vc Mean Difference - %.4f  StdDev - %.4f\\r\\n# Slope - %.4f Intercept - %.4f", w151, w116, w150, w149) -> (resulting string=w131:string)  [unwired: 2 in, 1 out]
            n131 = String To Path(string=w161) -> (path=w159:path)
            n132 = Format Into String(format string="# Hx-Vx Mean Difference - %.4f  StdDev - %.4f\\r\\n# Slope - %.4f Intercept - %.4f", w146, w117, w145, w144) -> (resulting string=w130:string)  [unwired: 2 in, 1 out]
            n133 = Build Array (concatenate)(w141, w140, w139, "# SigGen dBm   dbmHc      dbmHx      dbmVc      dbmVx", w126, w131, w130) -> (w155:string[])
            n134 = Write to Text File(file (use dialog)=w166, text=w155, error in=w165) -> (refnum out=w164:refnum<file>, error out=w163:errorcluster)  [unwired: 1 in, 1 out]
            n135 = Close File(refnum=w164, error in=w163) -> (path=w160:path)  [unwired: 1 out]
            n136 = Move(source path=w160, 10:w159) -> (3:→"Cal Output File":path)  [unwired: 3 in, 2 out]
          }
        }
        n137 = local write "C-State"(w113) -> ()
        n138 = property on="READY" class="Bool"("Visible"=w111) -> ()  [unwired: 2 in, 2 out]
      }
      frame "Stop" {
        # "Releasing the\nqueue stops\nthe consumer loop(s)."
        n139 = local write "C-State"(w244) -> ()
        n140 = property on="READY" class="Bool"("Visible"=w242) -> ()  [unwired: 2 in, 2 out]
        n141 = property on="Instructions" class="Str"("Visible"=w241) -> ()  [unwired: 2 in, 2 out]
        n142 = Release Queue(queue=w243) -> ()  [unwired: 2 in, 3 out]
      }
    }
  }
  n143 = while {
    tunnel: w10 -> [w249]
    tunnel: w8 -> [w248]
    stop <- w246 stop-if-true
    n144 = event shown="[5] \"Stop\": Value Change" {
      selector: _ -> [_ _ _ _ _ _ _]
      dyn-events: _ -> [_ _ _ _ _ _ _]
      timeout: 1000 -> [_ _ _ _ _ _ _]
      tunnel: w249 -> [w254 w259 w264 w269 w273 w277 w287]
      tunnel: w248 -> [w253 w258 w263 w268 w272 w279 w283]
      tunnel: [w252 w257 w262 w267 w271 w282 w285] -> _
      tunnel: [FALSE FALSE FALSE FALSE FALSE ("status") FALSE w286] -> w246
      event "Calibrate": Value Change {
        w250 = "Calibrate" ("element")
        n145 = event-data() -> ()  [unwired: 1 in, 1 out]
        n146 = local write "P-State"(w250) -> ()
        n147 = Enqueue Element(queue=w254, element=w250, error in (no error)=w253) -> (error out=w252:errorcluster)  [unwired: 1 in, 2 out]
      }
      event "Switches": Value Change {
        w255 = "Switches" ("element")
        n148 = event-data() -> ()  [unwired: 1 in, 1 out]
        n149 = local write "P-State"(w255) -> ()
        n150 = Enqueue Element(queue=w259, element=w255, error in (no error)=w258) -> (error out=w257:errorcluster)  [unwired: 1 in, 2 out]
      }
      event "121 dB": Value Change {
        w260 = "121 dB" ("element")
        n151 = event-data() -> ()  [unwired: 1 in, 1 out]
        n152 = local write "P-State"(w260) -> ()
        n153 = Enqueue Element(queue=w264, element=w260, error in (no error)=w263) -> (error out=w262:errorcluster)  [unwired: 1 in, 2 out]
      }
      event "70 dB": Value Change {
        w265 = "70 dB" ("element")
        n154 = event-data() -> ()  [unwired: 1 in, 1 out]
        n155 = local write "P-State"(w265) -> ()
        n156 = Enqueue Element(queue=w269, element=w265, error in (no error)=w268) -> (error out=w267:errorcluster)  [unwired: 1 in, 2 out]
      }
      event "Configuration 1": Value Change {
        w274 = "Configuration 1" ("element")
        n157 = event-data() -> ()  [unwired: 1 in, 3 out]
        n158 = local write "P-State"(w274) -> ()
        n159 = Enqueue Element(queue=w273, element=w274, error in (no error)=w272) -> (error out=w271:errorcluster)  [unwired: 1 in, 2 out]
      }
      event "Stop": Value Change {
        w280 = "Stop" ("element")
        n160 = event-data() -> ()  [unwired: 1 in, 1 out]
        n161 = Enqueue Element(queue=w277, element="Initialize", error in (no error)=w279) -> (queue out=w276:refnum<queue>, error out=w278:errorcluster)  [unwired: 1 in, 1 out]
        n162 = local write "P-State"(w280) -> ()
        n163 = Enqueue Element(queue=w276, element=w280, error in (no error)=w278) -> (error out=w282:errorcluster)  [unwired: 1 in, 2 out]
      }
      event Timeout {
        n164 = event-data() -> ()  [unwired: 1 in, 1 out]
        n165 = Get Queue Status(queue=w287, error in (no error)=w283) -> (error out=w285:errorcluster)  [unwired: 1 in, 7 out]
        n166 = Unbundle By Name(w285) -> ("status"=w286:bool)
        "P-State" <- "Timeout" ("element")
      }
    }
  }
  "Instructions" <- "drx calibration vi\n\n1 - Disable or turn off transmitter\n2 - Stow Antenna (point vertically)\n3 - Start the labview program by clicking the Run arrow\n     (left most button under  drop down menues)\n     start cycle time about 35 seconds\n3 - Wait for the red 'BUSY' light to change to green 'READY'\n     The 'active' controls on the control tab are the 'TsPring/TsGrabber'\n     and the 'Start dBm', 'Step Size' and 'Steps' controls \n4 - Calibrate with the red  'Calibrate' button\n      calibration cycle time is about 5 minutes\n5 - Calibration cycle can be aborted with the 'Abort Cal' button which\n     is visable only during the cal cycle\n6 - exit the program with the red 'EXIT' button\n      exit cycle time about 20 seconds\n\nHints:\nWait for the green 'READY' light before clicking buttons" ("String")
